vi "shift visible array up one.vi"(8 "error in (no error)":errorcluster, 11 "Array in":refnum<vi>) -> (0 "error out":errorcluster, 3 "Array out":refnum<vi>)   [LabVIEW 2013, in "PID Module editor node.lvclass"]
doc: "This VI shifts the visible array up one element"
uses:
  PID Module editor node.lvclass
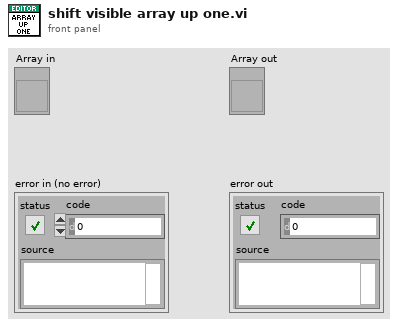
[diagram p1: front panel]
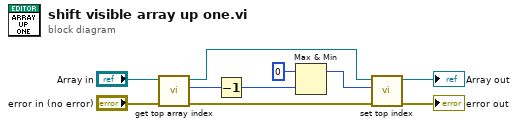
[diagram p0: block diagram]
diagram:
  n1 = call "get top array index.vi"("error in (no error)"="error in (no error)", "Array in"="Array in") -> ("error out"=w1:errorcluster, "top index"=w6:u32, "Array out"=w4:refnum<vi>)  [unwired: 6 in, 1 out]
  n2 = Decrement(x=w6) -> (x-1=w9:u32)
  n3 = Max & Min(x=u32 0 ("y"), y=w9) -> (max(x,y)=w5:u32)  [unwired: 1 out]
  n4 = call "set top index.vi"("error in (no error)"=w1, "Numeric"=w5, "Array in"=w4) -> ("error out"=→"error out":errorcluster, "Array out"=→"Array out":refnum<vi>)  [unwired: 7 in]
